vi "Parse SSH_FXP_DATA.vi"(8 "error in":errorcluster, 11 "payload":u8[](array[numeric])) -> (0 "error out":errorcluster, 3 "data":u8[](array[numeric]))   [LabVIEW 2020, in "NI_SFTP.lvlib"]
uses:
  <vilib>/net/SFTP/NI_SFTP.lvlib
  fe9cab8e-2cf0-3fe7-1c9b-f8983c6ade3f.vi
  <vilib>/Bit Manipulation/Network-Order Bytes To Words Poly.vi
  <vilib>/Bit Manipulation/wrappers/Network-Order Bytes To Words/Network-Order Bytes To Words U32.vi
  <vilib>/net/SFTP/Low Level Connection/Low Level Connection.lvclass
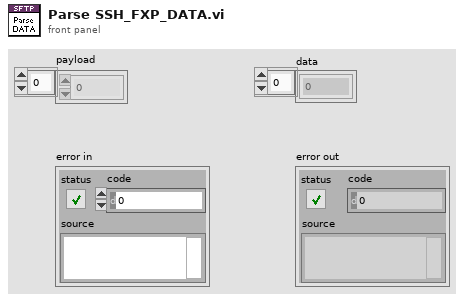
[diagram p1: front panel]
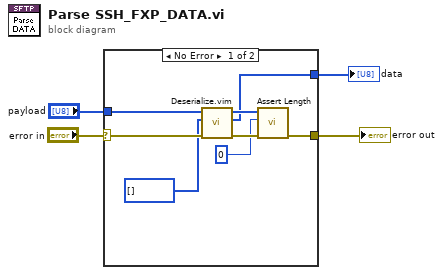
[diagram p0: block diagram]
diagram:
  n1 = case shown="No Error" "error in" {
    selector: "error in" -> [w11 w13]
    tunnel: [w8 w13] -> w3
    tunnel: "payload" -> [w12 _]
    tunnel: [w6 _] -> w1
    frame No Error {
      n2 = call "Deserialize.vim"("error in"=w11, "type"=u8[] [], "bytes"=w12) -> ("error out"=w9:errorcluster, "value"=w6:u8[], "remaining bytes"=w10:u8[])  [unwired: 6 in]
      n3 = call <vilib>:"Assert Length.vi"("error in"=w9, "asserted length"=u32 0, "string in"=w10) -> ("error out"=w8:errorcluster)  [unwired: 7 in, 1 out]
    }
    frame Error {
    }
  }
  "error out" <- w3
  "data" <- w1
